vi "08 LV - CSV Ingest.vi"() -> ()   [LabVIEW 2020]
uses:
  client/client.lvlib
  client/Client/Client.lvclass
  client/List/List.lvclass
  client/Channel/Channel.lvclass
  client/Dataset/Dataset.lvclass
  client/TabularIngestStaging/TabularIngestStaging.lvclass
panel:
  out "channel list":string[](array[string])
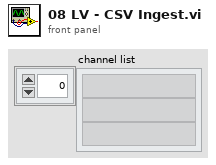
[diagram p1: front panel]
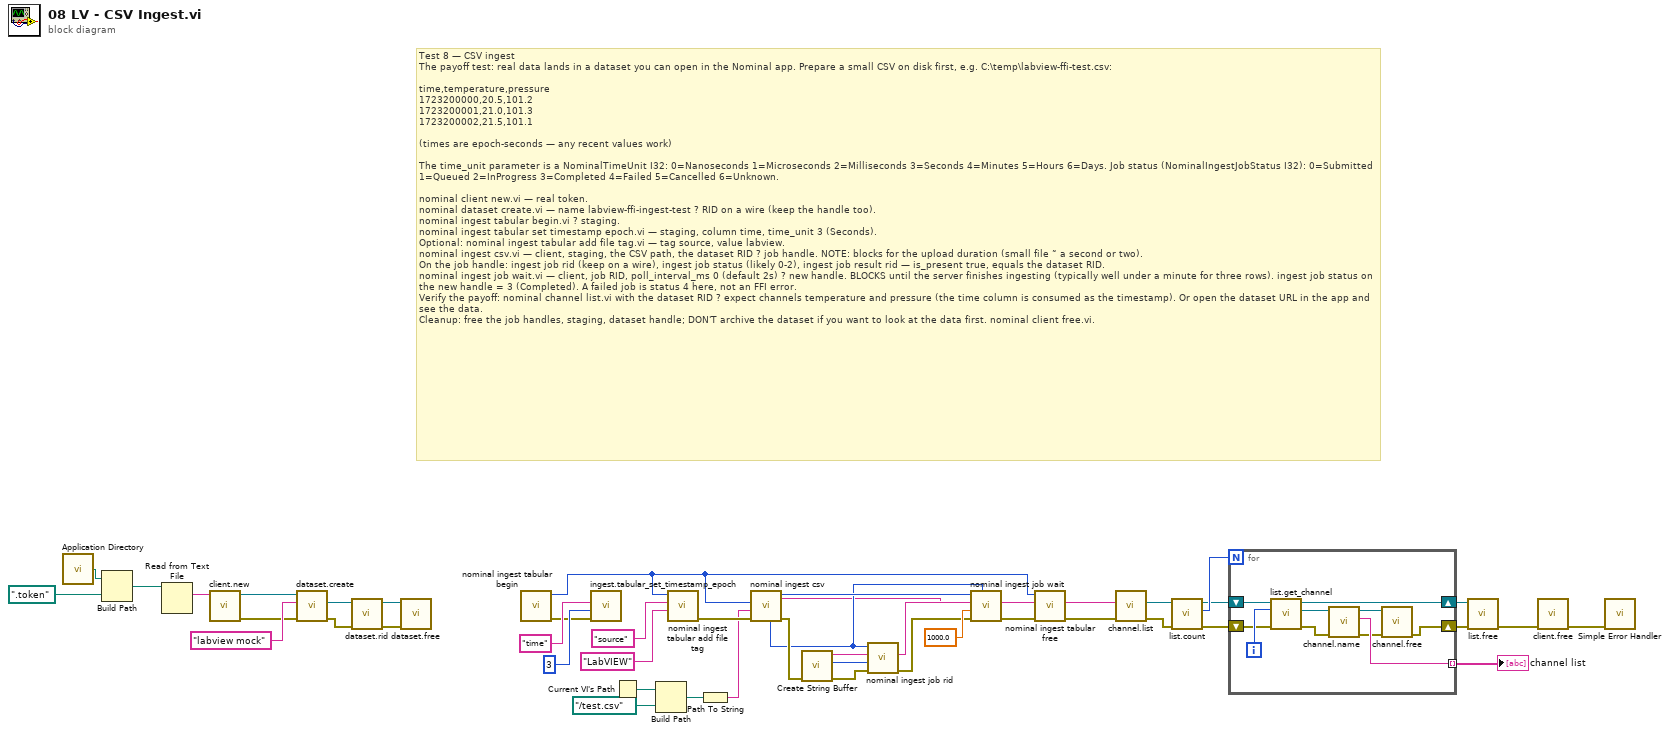
[diagram p0: block diagram]
diagram:
  # "Test 8 — CSV ingest\nThe payoff test: real data lands in a dataset you can open in the Nominal app. Prepare a small CSV on disk first, e.g. C:\\temp\\labview-ffi-test.csv:\n\ntime,temperature,pressure\n1723200000,20.5,101.2\n1723200001,21.0,101.3\n1723200002,21.5,101.1\n\n(times are epoch-seconds — any recent values work)\n\nThe time_unit parameter is a NominalTimeUnit I32: 0=Nanoseconds 1=Microseconds 2=Milliseconds 3=Seconds 4=Minutes 5=Hours 6=Days. Job status (NominalIngestJobStatus I32): 0=Submitted 1=Queued 2=InProgress 3=Completed 4=Failed 5=Cancelled 6=Unknown.\n\nnominal client new.vi — real token.\nnominal dataset create.vi — name labview-ffi-ingest-test ? RID on a wire (keep the handle too).\nnominal ingest tabular begin.vi ? staging.\nnominal ingest tabular set timestamp epoch.vi — staging, column time, time_unit 3 (Seconds).\nOptional: nominal ingest tabular add file tag.vi — tag source, value labview.\nnominal ingest csv.vi — client, staging, the CSV path, the dataset RID ? job handle. NOTE: blocks for the upload duration (small file ˜ a second or two).\nOn the job handle: ingest job rid (keep on a wire), ingest job status (likely 0-2), ingest job result rid — is_present true, equals the dataset RID.\nnominal ingest job wait.vi — client, job RID, poll_interval_ms 0 (default 2s) ? new handle. BLOCKS until the server finishes ingesting (typically well under a minute for three rows). ingest job status on the new handle = 3 (Completed). A failed job is status 4 here, not an FFI error.\nVerify the payoff: nominal channel list.vi with the dataset RID ? expect channels temperature and pressure (the time column is consumed as the timestamp). Or open the dataset URL in the app and see the data.\nCleanup: free the job handles, staging, dataset handle; DON'T archive the dataset if you want to look at the data first. nominal client free.vi."
  n1 = call <vilib>:"Application Directory.vi"() -> ("Application Directory"=w45:path)
  n2 = Build Path(base path=w45, name or relative path=path ".token") -> (appended path=w43:path)
  n3 = Read from Text File(file (use dialog)=w43) -> (text=w11:string)  [unwired: 3 in, 3 out]
  n4 = call "client.new.vi"("token"=w11) -> ("error out"=w8:errorcluster, "Client out"=w10:refnum<class "Client.lvclass">)  [unwired: 9 in]
  n5 = call "dataset.create.vi"("error in"=w8, "name"="labview mock", "Client in"=w10) -> ("error out"=w6:errorcluster, "Dataset"=w7:refnum<class "Dataset.lvclass">)  [unwired: 6 in, 1 out]
  n6 = call "dataset.rid.vi"("error in"=w6, "Dataset in"=w7) -> ("error out"=w4:errorcluster, "Dataset out"=w5:refnum<class "Dataset.lvclass">)  [unwired: 7 in, 1 out]
  n7 = call "dataset.free.vi"("error in"=w4, "Dataset"=w5) -> ()  [unwired: 9 in, 1 out]
  n8 = call "nominal ingest tabular begin.vi"() -> ("error out"=w1:errorcluster, "out_staging out"=w31:i32)  [unwired: 9 in, 1 out]
  n9 = call "ingest.tabular_set_timestamp_epoch.vi"("error in"=w1, "time unit"=3 ("time_unit"), "column"="time") -> ()  [unwired: 7 in, 2 out]
  n10 = Current VI's Path() -> (path=w38:path)
  n11 = Build Path(base path=w38, name or relative path=path "../test.csv") -> (appended path=w36:path)
  n12 = call "nominal ingest tabular add file tag.vi"("value"="LabVIEW" ("tag"), "tag"="source", "staging"=w31) -> ("error out"=w39:errorcluster, "error in (no error)"=w40:errorcluster)  [unwired: 6 in, 1 out]
  n13 = Path To String(path=w36) -> (string=w35:string)
  n14 = call "nominal ingest csv.vi"("error in (no error)"=w39, "file_path"=w35, "staging"=w31) -> ("error out"=w28:errorcluster, "out_job out"=w23:i32, "dataset_rid"=w22:string, "client"=w33:i32)  [unwired: 4 in, 1 out]
  n15 = call "Create String Buffer.vi"("error in"=w28) -> ("error out"=w29:errorcluster, "dub Buffer Size"=w24:i32, "String Buffer"=w30:string)  [unwired: 8 in]
  n16 = call "nominal ingest job rid.vi"("error in (no error)"=w29, "cap"=w24, "buf"=w30, "job"=w23) -> ("error out"=w26:errorcluster, "buf out"=w27:string)  [unwired: 4 in, 2 out]
  n17 = call "nominal ingest job wait.vi"("out_job"=w23, "error in (no error)"=w26, "poll_interval_ms"=1000.0, "rid"=w27, "client"=w33) -> ("error out"=w25:errorcluster)  [unwired: 4 in, 2 out]
  n18 = call "nominal ingest tabular free.vi"("error in (no error)"=w25, "staging"=w31) -> ("error out"=w21:errorcluster)  [unwired: 8 in, 1 out]
  n19 = call "channel.list.vi"("error in"=w21, "data source rid"=w22) -> ("error out"=w19:errorcluster, "List"=w20:refnum<class "List.lvclass">)  [unwired: 7 in, 1 out]
  n20 = call "list.count.vi"("error in"=w19, "List in"=w20) -> ("error out"=w18:errorcluster, "count"=w17:u32, "List out"=w16:refnum<class "List.lvclass">)  [unwired: 7 in]
  n21 = for {
    N: w17 -> [_]
    shift-right: [w47] -> w14
    shift-left: w18 -> [w51]
    tunnel: [w55] -> w32 mode=indexing
    shift-right: [w46] -> w15
    shift-left: w16 -> [w50]
    i -> [w54]
    n22 = call "list.get_channel.vi"("error in (no error)"=w51, "index"=w54, "List in"=w50) -> ("error out"=w52:errorcluster, "Channel"=w53:refnum<class "Channel.lvclass">, "List out"=w46:refnum<class "List.lvclass">)  [unwired: 6 in]
    n23 = call "channel.name.vi"("error in"=w52, "Channel in"=w53) -> ("error out"=w48:errorcluster, "name"=w55:string, "Channel out"=w49:refnum<class "Channel.lvclass">)  [unwired: 7 in]
    n24 = call "channel.free.vi"("error in"=w48, "Channel"=w49) -> ("error out"=w47:errorcluster)  [unwired: 9 in]
  }
  "channel list" <- w32
  n25 = call "list.free.vi"("error in"=w14, "List in"=w15) -> ("error out"=w12:errorcluster)  [unwired: 9 in]
  n26 = call "client.free.vi"("error in"=w12) -> ("error out"=w13:errorcluster)  [unwired: 10 in]
  n27 = call <vilib>:"Simple Error Handler.vi"("error in (no error)"=w13) -> ()  [unwired: 4 in, 5 out]
